vi "Close Vecto.vi"(8 "error in (no error)":errorcluster, 11 "Volatus Core in":refnum<class "Volatus Core.lvclass">) -> (0 "error out":errorcluster, 3 "Volatus Core out":refnum<class "Volatus Core.lvclass">)   [LabVIEW 2020, in "Volatus.lvlib" / "Volatus Core.lvclass"]
uses:
  Volatus Core.lvclass
  C:/dev/lv20CE/relink/lv-volatus/Volatus/Module/Module.lvclass
  Reload State.ctl
  Module/Module.lvclass/Module.ctl
  Volatus Core.lvclass/Volatus Core.ctl
  Module/Module.lvclass
  lv-vecto/Vecto/Vecto/Vecto.lvclass
  VolatusAPI/VolatusAPI.lvclass
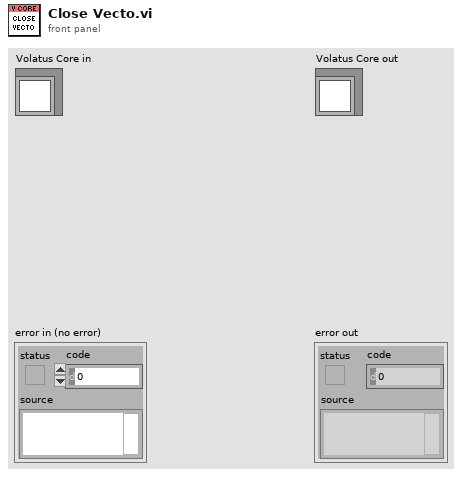
[diagram p1: front panel]
types:
  T1 = typedef "Volatus.lvlib/Volatus Core.lvclass/Reload State.ctl" = enum16{"None", "Stop Modules", "Close Vecto", "Reload", "Restart"}
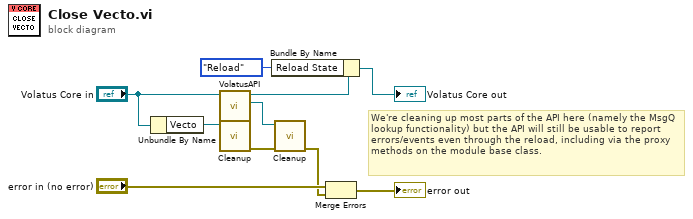
[diagram p0: block diagram]
diagram:
  # "We're cleaning up most parts of the API here (namely the MsgQ lookup functionality) but the API will still be usable to report errors/events even through the reload, including via the proxy methods on the module base class."
  n1 = Unbundle By Name("Volatus Core in") -> ("Vecto"=w9:refnum<class "Vecto.lvclass">)
  n2 = call "VolatusAPI.vi"("Module in"="Volatus Core in") -> ("VolatusAPI"=w7:refnum<class "VolatusAPI.lvclass">, "Module out"=w5:refnum<class "Volatus Core.lvclass">)  [unwired: 9 in]
  n3 = call "Cleanup.vi"("Vecto in"=w9) -> ("error out"=w8:errorcluster)  [unwired: 10 in]
  n4 = Bundle By Name(cluster=w5, "Reload State"=Reload_State."Reload") -> (→"Volatus Core out":refnum<class "Volatus Core.lvclass">)
  n5 = call-dynamic "Cleanup.vi"("error in (no error)"=w8, "VolatusAPI in"=w7) -> ("error out"=w3:errorcluster)  [unwired: 9 in]
  n6 = Merge Errors("error in (no error)", w3) -> (→"error out":errorcluster)
